vi "ClawSetOpenClose.vi"(11 "Open?":bool) -> ()   [LabVIEW 2020]
uses:
  ClawGlobal.vi
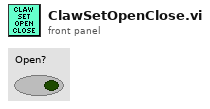
[diagram p1: front panel]
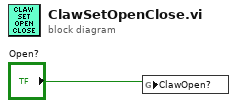
[diagram p0: block diagram]
diagram:
  n1 = global write "ClawGlobal.vi" "ClawOpen?"("Open?") -> ()
